vi "PIC7-DEMO.vi"() -> ()   [LabVIEW 2016]
panel:
  in  "text":string
  in  "alignment(left, top)":T1
  in  "origin":cluster{"x":i16, "y":i16}
  out "Shadow":u32(colorbox)=143
  out "Hilite":u32(colorbox)=5000411
  in  "Percentage(30)":dbl=30.0 format="%0.2f"
  in  "Color In":u32(colorbox)=204
  out "new picture":picture
  in  "line endpoints":cluster{"x":i16, "y":i16}[](array[cluster])
  in  "color(black)":u32(colorbox)
  in  "fill?(F)":bool
  in  "rect":T2
  in  "end point":cluster{"x":i16, "y":i16}
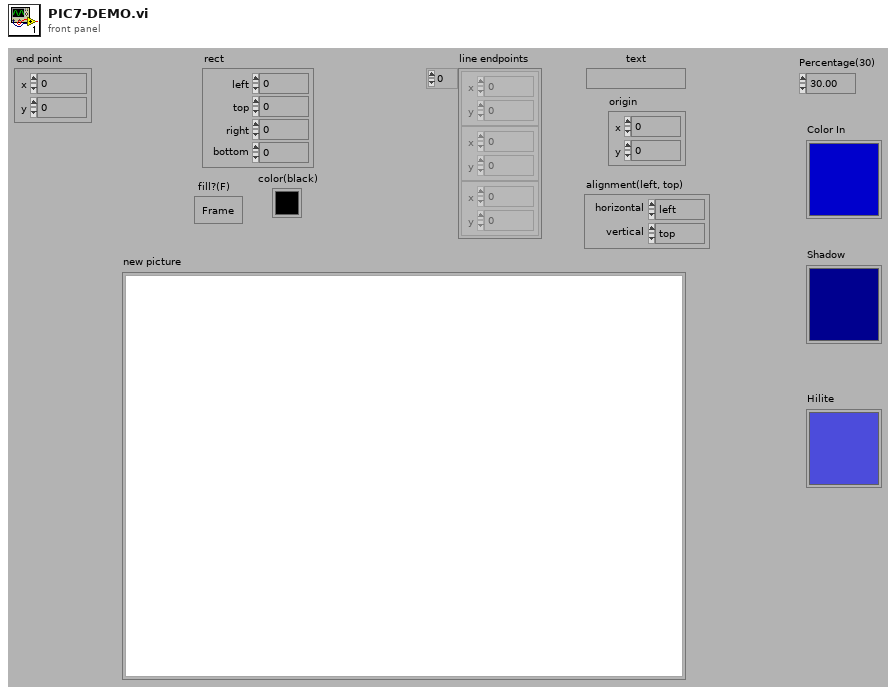
[diagram p1: front panel]
types:
  T1 = cluster{"horizontal":enum16{"left", "center", "right"}, "vertical":enum16{"top", "center", "bottom"}}
  T2 = cluster{"left":i16, "top":i16, "right":i16, "bottom":i16}
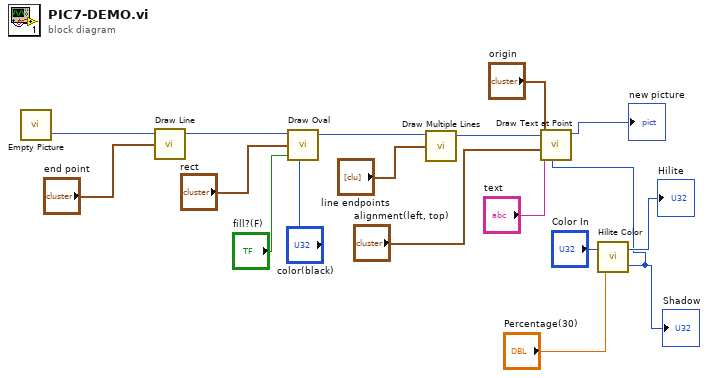
[diagram p0: block diagram]
diagram:
  n1 = call "Empty Picture"() -> ("empty picture"=w17:picture)
  n2 = call <vilib>:"Draw Line.vi"("picture"=w17, "end point"="end point") -> ("new picture"=w15:picture)  [unwired: 7 in]
  n3 = call <vilib>:"Draw Oval.vi"("picture"=w15, "rect"="rect", "fill?(F)"="fill?(F)", "color(black)"="color(black)") -> ("new picture"=w11:picture)  [unwired: 5 in]
  n4 = call <vilib>:"Draw Multiple Lines.vi"("picture"=w11, "line endpoints"="line endpoints") -> ("new picture"=w7:picture)  [unwired: 7 in]
  n5 = call <vilib>:"Hilite Color.vi"("Percentage(30)"="Percentage(30)", "Color In"="Color In") -> ("Shadow"=w1:u32, "Hilite"=→"Hilite":u32)
  "Shadow" <- w1
  n6 = call <vilib>:"Draw Text at Point.vi"("text color(black)"=w1, "text"="text", "alignment(left, top)"="alignment(left, top)", "origin"="origin", "picture"=w7) -> ("new picture"=→"new picture":picture)  [unwired: 5 in, 1 out]
